vi "PPR_TRAJECTORY_EXECUTE_ABS.vi"(8 "Init":bool, 10 "Max Wheel Speed M/S":dbl, 11 "End Pose ENG":T6={"TRANSLATION"={"X"=0.0, "Y"=0.0}, "ROTATION"={"VALUE"=0.0, "COS"=1.0, "SIN"=0.0}} {"ROTATION"."SIN" format="%13.4f"; "ROTATION"."COS" format="%13.4f"; "ROTATION"."VALUE" format="%13.4f"; "TRANSLATION"."Y" format="%14.3f"; "TRANSLATION"."X" format="%14.3f"}) -> (0 "AtReference":bool, 2 "Right Speed Dmd M/S":dbl, 3 "Left Speed Dmd M/S":dbl)   [LabVIEW 2019]
uses:
  <vilib>/Rock Robotics/WPI/ThirdParty/JAS_Junk/TrajLib/TypeDef/POSE2D.ctl
  <vilib>/Rock Robotics/WPI/ThirdParty/JAS_Junk/TrajLib/TypeDef/TRANSLATION2D.ctl
  <vilib>/Rock Robotics/WPI/ThirdParty/JAS_Junk/TrajLib/TypeDef/ROTATION2D.ctl
  <vilib>/Rock Robotics/WPI/ThirdParty/MJansen/PathPlanner/TypeDef/PathPlannerTrajectory.ctl
  <vilib>/Rock Robotics/WPI/ThirdParty/MJansen/PathPlanner/TypeDef/PathPlannerTrajectoryState.ctl
  <vilib>/Rock Robotics/WPI/ThirdParty/MJansen/PathPlanner/TypeDef/PathPlannerPathConstraints.ctl
  <vilib>/Rock Robotics/WPI/ThirdParty/JAS_Junk/TrajLib/VI/Util_GetTime_U32.vi
  <vilib>/Rock Robotics/WPI/ThirdParty/JAS_Junk/TrajLib/Rotation2d_UnaryMinus.vi
  <vilib>/Rock Robotics/WPI/ThirdParty/JAS_Junk/TrajLib/Rotation2d_RotateBy.vi
  <vilib>/Rock Robotics/WPI/ThirdParty/JAS_Junk/TrajLib/Rotation2d_GetRadians.vi
  <vilib>/Rock Robotics/WPI/ThirdParty/JAS_Junk/TrajLib/Rotation2d_CreateAngle.vi
  <vilib>/Rock Robotics/WPI/ThirdParty/JAS_Junk/TrajLib/Rotation2d_CreateXY.vi
  <vilib>/Rock Robotics/WPI/ThirdParty/JAS_Junk/TrajLib/Util_CalcDist.vi
  <vilib>/Rock Robotics/WPI/ThirdParty/JAS_Junk/TrajLib/VI/Util_GetTime_U64.vi
  PPR_TRAJECTORY_GLOBALS.vi
  Diff_Drive_System/PPR_DRIVE_GLOBALS.vi
  <vilib>/Rock Robotics/WPI/ThirdParty/JAS_Junk/TrajLib/Trajectory_Library.lvlib
  <vilib>/Rock Robotics/WPI/ThirdParty/MJansen/PathPlanner/PathPlanner24.lvlib
panel:
  out "Position Error M":dbl
  out "PathPlannerTrajectory":T1 {"States"."TargetHolonomicRotation"."SIN" format="%13.4f"; "States"."TargetHolonomicRotation"."COS" format="%13.4f"; "States"."TargetHolonomicRotation"."VALUE" format="%13.4f"; "States"."Heading"."SIN" format="%13.4f"; "States"."Heading"."COS" format="%13.4f"; "States"."Heading"."VALUE" format="%13.4f"; "States"."PositionMeters"."Y" format="%14.3f"; "States"."PositionMeters"."X" format="%14.3f"}
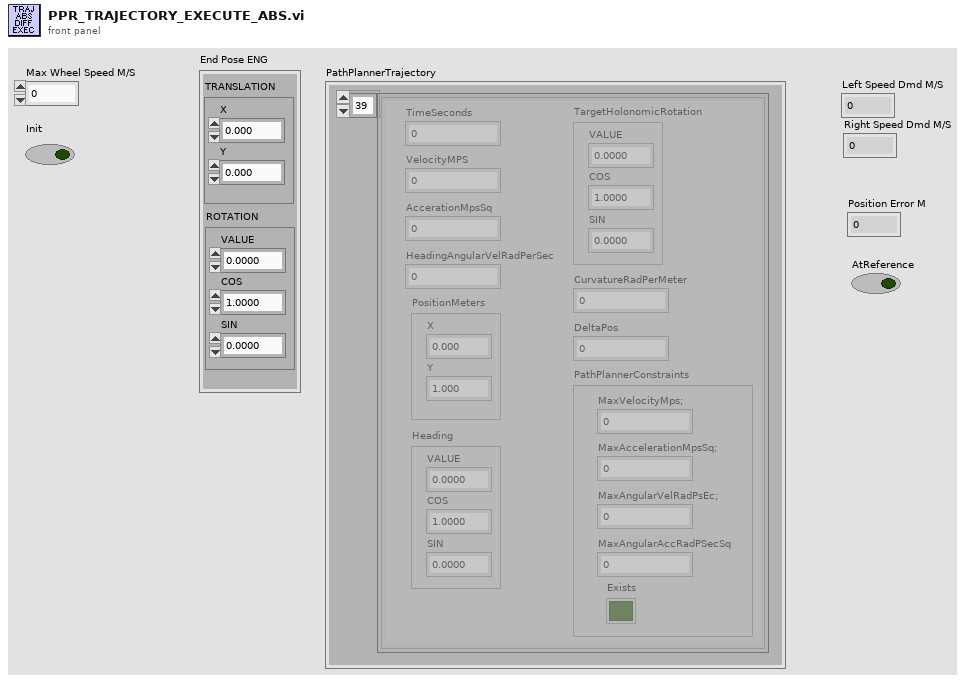
[diagram p1: front panel]
types:
  T1 = typedef "PathPlanner24.lvlib/PathPlannerTrajectory.ctl" = cluster{"States":T2[]}
  T2 = typedef "PathPlanner24.lvlib/PathPlannerTrajectoryState.ctl" = cluster{"TimeSeconds":dbl, "VelocityMPS":dbl, "AccerationMpsSq":dbl, "HeadingAngularVelRadPerSec":dbl, "PositionMeters":T3, "Heading":T4, "TargetHolonomicRotation":T4, "CurvatureRadPerMeter":dbl, "PathPlannerConstraints":T5, "DeltaPos":dbl}
  T3 = typedef "Trajectory_Library.lvlib/TRANSLATION2D.ctl" = cluster{"X":dbl, "Y":dbl}
  T4 = typedef "Trajectory_Library.lvlib/ROTATION2D.ctl" = cluster{"VALUE":dbl, "COS":dbl, "SIN":dbl}
  T5 = typedef "PathPlanner24.lvlib/PathPlannerPathConstraints.ctl" = cluster{"MaxVelocityMps;":dbl, "MaxAccelerationMpsSq;":dbl, "MaxAngularVelRadPsEc;":dbl, "MaxAngularAccRadPSecSq":dbl, "Exists":bool}
  T6 = typedef "Trajectory_Library.lvlib/POSE2D.ctl" = cluster{"TRANSLATION":T3, "ROTATION":T4}
  T7 = typedef "Trajectory_Library.lvlib/DIFF_DRIVE_KINEMATICS.ctl" = cluster{"TrackWidth_Meters":dbl}
  T8 = typedef "Trajectory_Library.lvlib/RAMSETE_EXE_TUNING.ctl" = cluster{"B":dbl, "Zeta":dbl, "X Tolerance M":dbl, "Y Tolerance M":dbl, "Heading Tolerance RAD":dbl, "Track Width M":dbl, "Max Speed M/S":dbl}
  T9 = typedef "Trajectory_Library.lvlib/RAMSETE.ctl" = cluster{"B":dbl, "Zeta":dbl, "poseTolerance":T6, "poseError":T6, "Enabled":bool}
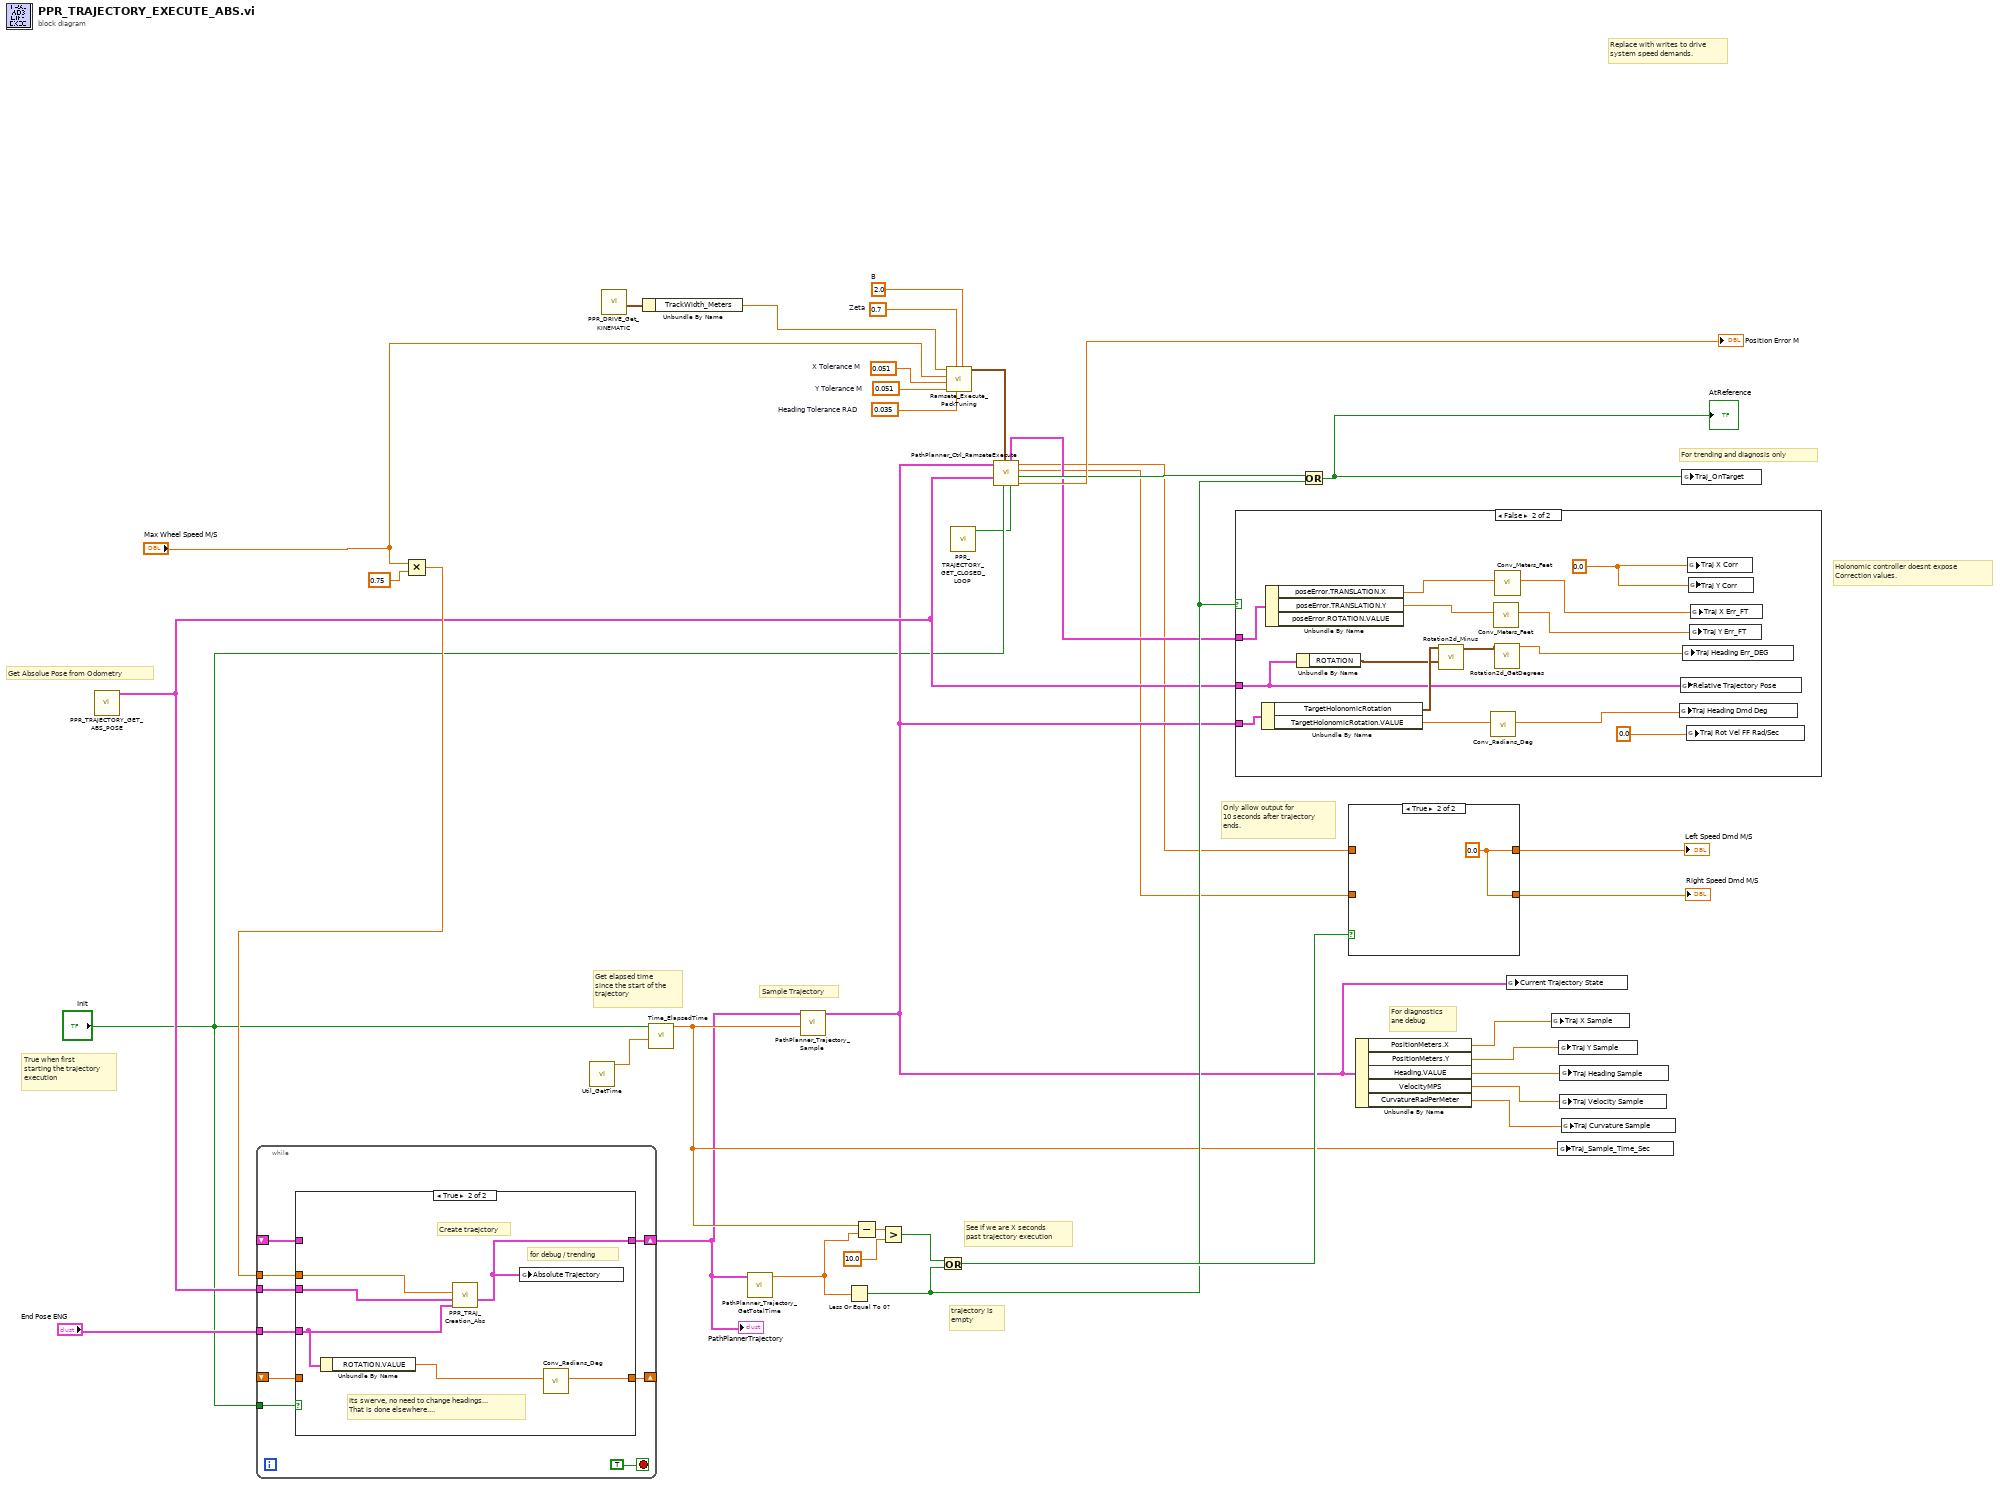
[diagram p0: block diagram]
diagram:
  w14 = 0.051  # X Tolerance M
  w15 = 0.051  # Y Tolerance M
  w16 = 0.7  # Zeta
  w17 = 0.035  # Heading Tolerance RAD
  w18 = 2.0  # B
  # "Replace with writes to drive\nsystem speed demands."
  # "trajectory is \nempty"
  # "True when first\nstarting the trajectory\nexecution"
  # "Get elapsed time\nsince the start of the\ntrajectory"
  # "Holonomic controller doesnt expose\nCorrection values."
  # "For trending and diagnosis only"
  # "For diagnostics\nane debug"
  # "Get Absolue Pose from Odometry"
  # "Sample Trajectory"
  # "See if we are X seconds \npast trajectory execution"
  # "Only allow output for\n10 seconds after trajectory\nends."
  n1 = call "PPR_TRAJECTORY_GET_ABS_POSE.vi"() -> ("Absolute Odometry Pose"=w13:T6)  [unwired: 11 in]
  n2 = Multiply(x="Max Wheel Speed M/S", y=0.75) -> (x*y=w22:dbl)
  n3 = while {
    tunnel: "Init" -> [w46]
    tunnel: w13 -> [w45]
    shift-right: [w44] -> w24
    shift-left: _ -> [w43]
    shift-right: [w42] -> _
    shift-left: _ -> [w41]
    tunnel: "End Pose ENG" -> [w40]
    tunnel: w22 -> [w39]
    stop <- TRUE stop-if-true
    n4 = case shown="True" w46 {
      tunnel: w45 -> [_ w51]
      tunnel: [w49 w52] -> w44
      tunnel: w43 -> [w49 _]
      tunnel: [w48 w54] -> w42
      tunnel: w41 -> [w48 _]
      tunnel: w40 -> [_ w55]
      tunnel: w39 -> [_ w50]
      frame False {
      }
      frame True {
        # "for debug / trending"
        # "Its swerve, no need to change headings...\nThat is done elsewhere...."
        # "Create traejctory"
        n5 = Unbundle By Name(w55) -> ("ROTATION.VALUE"=w53:dbl)
        n6 = call "PPR_TRAJ_Creation_Abs.vi"("End Pose  ENG"=w55, "Current Pose SI"=w51, "Max Velocity M/S"=w50) -> ("PathPlannerTrajectory"=w52:T1)  [unwired: 6 in, 2 out]
        n7 = global write "PPR_TRAJECTORY_GLOBALS.vi" "Absolute Trajectory"(w52) -> ()
        n8 = call <vilib>:"Conv_Radians_Deg.vi"("Radians"=w53) -> ("Degrees"=w54:dbl)  [unwired: 10 in]
      }
    }
  }
  "PathPlannerTrajectory" <- w24
  n9 = call <vilib>:"Util_GetTime.vi"() -> ("FPGA_Time_Seconds"=w36:dbl)  [unwired: 9 in, 2 out]
  n10 = call "PPR_DRIVE_Get_KINEMATIC.vi"() -> ("out DIFF_DRIVE_KINEMATICS"=w8:T7)  [unwired: 11 in]
  n11 = Unbundle By Name(w8) -> ("TrackWidth_Meters"=w7:dbl)
  n12 = call <vilib>:"Time_ElapsedTime.vi"("PassthroughTime_SEC"=w36, "Reset"="Init") -> ("Elapsed Time Sec"=w25:dbl)  [unwired: 9 in]
  n13 = call <vilib>:"PathPlanner_Trajectory_GetTotalTime.vi"("PathPlannerTrajectory"=w24) -> ("TotalTimeSeconds"=w23:dbl)  [unwired: 10 in]
  n14 = call <vilib>:"PathPlanner_Trajectory_Sample.vi"("Time"=w25, "PathPlannerTrajectory"=w24) -> ("PathPlannerState"=w12:T2)  [unwired: 9 in]
  n15 = Less Or Equal To 0?(x=w23) -> (x <= 0?=w26:bool)
  n16 = Subtract(x=w25, y=w23) -> (x-y=w38:dbl)
  n17 = Greater?(x=w38, y=10.0) -> (0:w29:bool)
  n18 = Or(x=w29, y=w26) -> (x .or. y?=w28:bool)
  n19 = call <vilib>:"Ramsete_Execute_PackTuning.vi"("B"=w18, "Heading Tolerance RAD"=w17, "Zeta"=w16, "Y Tolerance M"=w15, "X Tolerance M"=w14, "Max Speed M/S"="Max Wheel Speed M/S", "Track Width M"=w7) -> ("RAMSETE_EXE_TUNING"=w19:T8)  [unwired: 4 in]
  n20 = call "PPR_TRAJECTORY_GET_CLOSED_LOOP.vi"() -> ("AUTO_CLOSED_LOOP"=w10:bool)  [unwired: 11 in]
  n21 = call <vilib>:"PathPlanner_Ctrl_RamseteExecute.vi"("Enabled"=w10, "Reset"="Init", "RAMSETE_EXE_TUNING SI"=w19, "Current Pose SI"=w13, "PathPlannerState"=w12) -> ("Position Error M"=→"Position Error M":dbl, "At Reference"=w9:bool, "Right Speed Dmd M/S"=w3:dbl, "Left Speed Dmd M/S"=w5:dbl, "outRAMSETE"=w6:T9)  [unwired: 2 in]
  n22 = case shown="False" w26 {
    tunnel: w13 -> [_ w59]
    tunnel: w6 -> [_ w66]
    tunnel: w12 -> [_ w63]
    frame True {
    }
    frame False {
      w70 = 0.0 ("Y Corr")
      n23 = Unbundle By Name(w63) -> ("TargetHolonomicRotation"=w60:T4, "TargetHolonomicRotation.VALUE"=w62:dbl)
      n24 = Unbundle By Name(w66) -> ("poseError.TRANSLATION.X"=w65:dbl, "poseError.TRANSLATION.Y"=w64:dbl)  [unwired: 1 out]
      n25 = Unbundle By Name(w59) -> ("ROTATION"=w58:T4)
      n26 = call <vilib>:"Rotation2d_Minus.vi"("other ROTATION"=w58, "in ROTATION"=w60) -> ("out ROTATION"=w57:T4)  [unwired: 9 in]
      n27 = call <vilib>:"Conv_Radians_Deg.vi"("Radians"=w62) -> ("Degrees"=w61:dbl)  [unwired: 10 in]
      n28 = call <vilib>:"Conv_Meters_Feet.vi"("Meters"=w64) -> ("Feet"=w69:dbl)  [unwired: 10 in]
      n29 = call <vilib>:"Rotation2d_GetDegrees.vi"("in ROTATION"=w57) -> ("AngleDegrees"=w56:dbl)  [unwired: 10 in]
      n30 = call <vilib>:"Conv_Meters_Feet.vi"("Meters"=w65) -> ("Feet"=w68:dbl)  [unwired: 10 in]
      n31 = global write "PPR_TRAJECTORY_GLOBALS.vi" "Traj Heading Dmd Deg"(w61) -> ()
      n32 = global write "PPR_TRAJECTORY_GLOBALS.vi" "Relative Trajectory Pose"(w59) -> ()
      n33 = global write "PPR_TRAJECTORY_GLOBALS.vi" "Traj Heading Err_DEG"(w56) -> ()
      n34 = global write "PPR_TRAJECTORY_GLOBALS.vi" "Traj Rot Vel FF Rad/Sec"(0.0 ("Traj Heading Dmd Deg")) -> ()
      n35 = global write "PPR_TRAJECTORY_GLOBALS.vi" "Traj X Corr"(w70) -> ()
      n36 = global write "PPR_TRAJECTORY_GLOBALS.vi" "Traj Y Corr"(w70) -> ()
      n37 = global write "PPR_TRAJECTORY_GLOBALS.vi" "Traj Y Err_FT"(w69) -> ()
      n38 = global write "PPR_TRAJECTORY_GLOBALS.vi" "Traj X Err_FT"(w68) -> ()
    }
  }
  n39 = Or(x=w9, y=w26) -> (x .or. y?=w27:bool)
  "AtReference" <- w27
  n40 = case shown="True" w28 {
    tunnel: w5 -> [w72 _]
    tunnel: [w72 w73] -> w4
    tunnel: w3 -> [w71 _]
    tunnel: [w71 w73] -> w2
    frame False {
    }
    frame True {
      w73 = 0.0 ("vX")
    }
  }
  "Left Speed Dmd M/S" <- w4
  "Right Speed Dmd M/S" <- w2
  n41 = Unbundle By Name(w12) -> ("PositionMeters.X"=w35:dbl, "PositionMeters.Y"=w34:dbl, "Heading.VALUE"=w33:dbl, "VelocityMPS"=w32:dbl, "CurvatureRadPerMeter"=w31:dbl)
  n42 = global write "PPR_TRAJECTORY_GLOBALS.vi" "Current Trajectory State"(w12) -> ()
  n43 = global write "PPR_TRAJECTORY_GLOBALS.vi" "Traj X Sample"(w35) -> ()
  n44 = global write "PPR_TRAJECTORY_GLOBALS.vi" "Traj_Sample_Time_Sec"(w25) -> ()
  n45 = global write "PPR_TRAJECTORY_GLOBALS.vi" "Traj Y Sample"(w34) -> ()
  n46 = global write "PPR_TRAJECTORY_GLOBALS.vi" "Traj Heading Sample"(w33) -> ()
  n47 = global write "PPR_TRAJECTORY_GLOBALS.vi" "Traj Velocity Sample"(w32) -> ()
  n48 = global write "PPR_TRAJECTORY_GLOBALS.vi" "Traj Curvature Sample"(w31) -> ()
  n49 = global write "PPR_TRAJECTORY_GLOBALS.vi" "Traj_OnTarget"(w27) -> ()
